vi "Turn To Angle Teleop.vi"(8 "Z Axis":dbl, 9 "PID gains":T1={"proportional gain (Kc)"=0.035, "integral time (Ti, min)"=0.0, "derivative time (Td, min)"=0.0018}, 10 "POV":i16, 11 "output range":cluster{"output high":dbl, "output low":dbl}={"output high"=1.0, "output low"=-1.0}) -> (2 "Adjustment Voltage":dbl)   [LabVIEW 2018]
uses:
  <vilib>/addons/control/pid/pid.llb/PID (DBL).vi
  <vilib>/addons/control/pid/NI_PID_pid.lvlib
panel:
  # ".0202"
  # "0"
  # ".0032150"
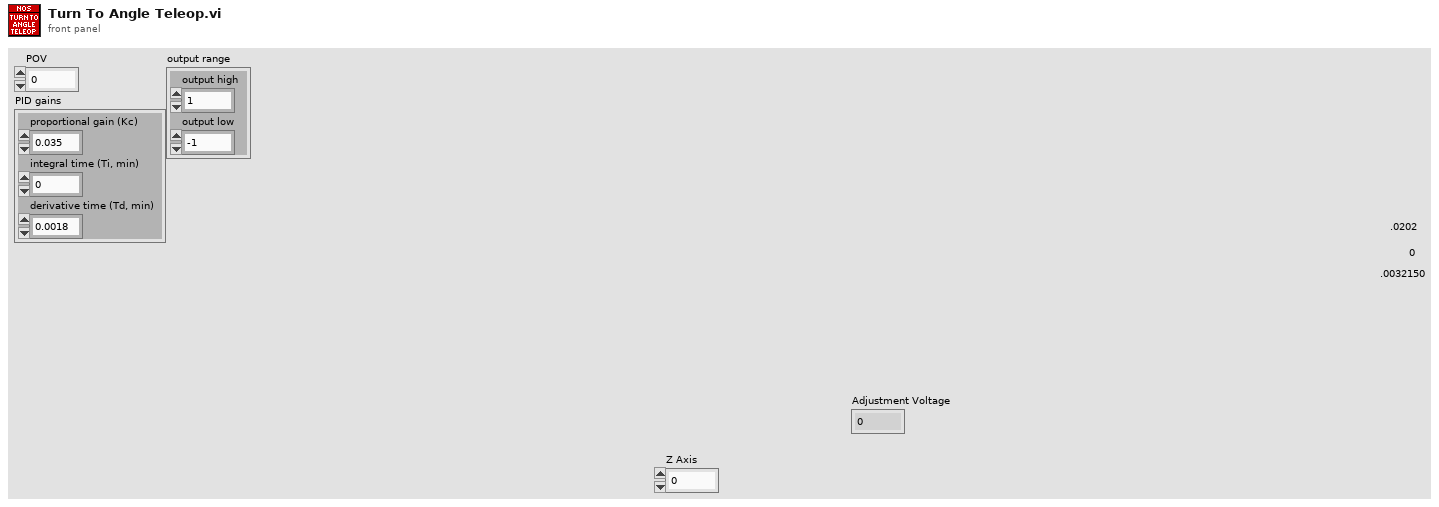
[diagram p1: front panel]
types:
  T1 = cluster{"proportional gain (Kc)":dbl, "integral time (Ti, min)":dbl, "derivative time (Td, min)":dbl}
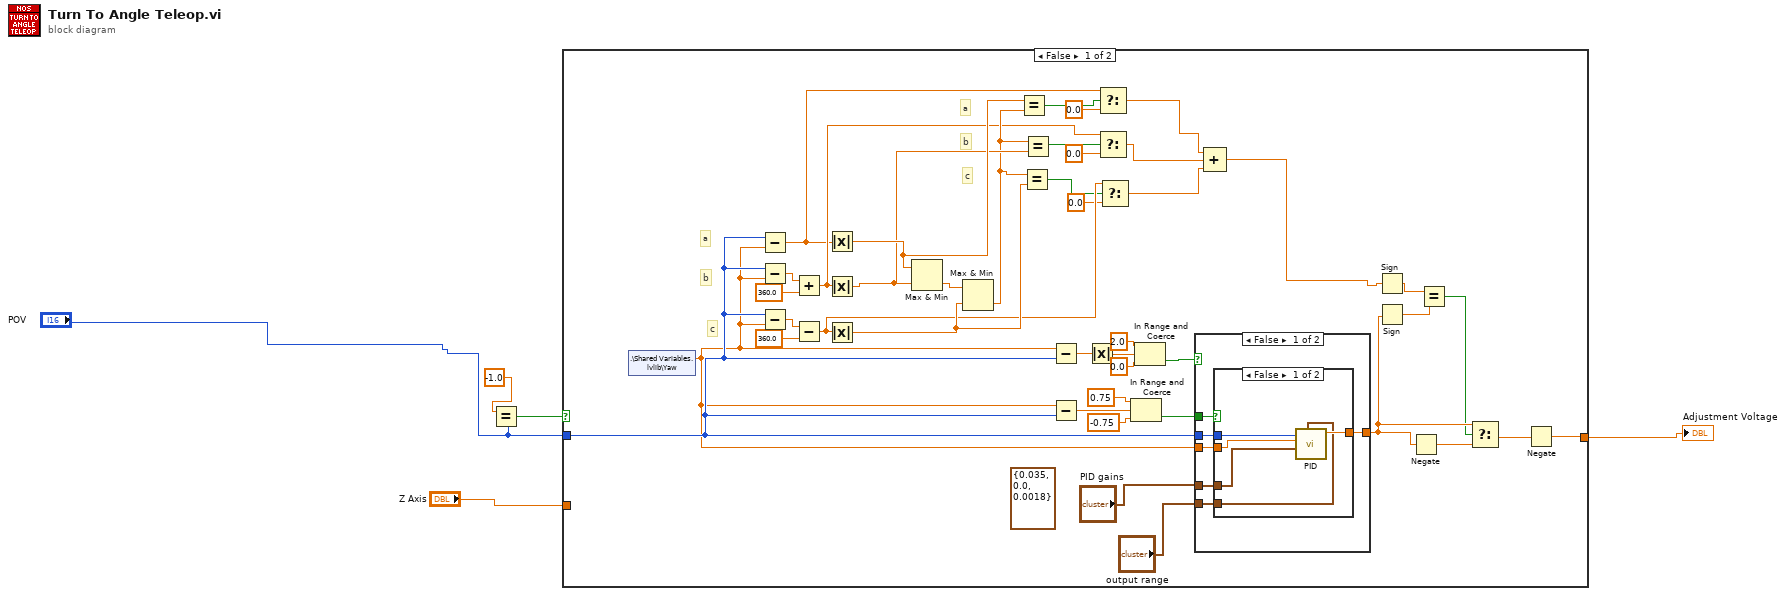
[diagram p0: block diagram]
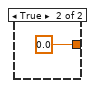
[diagram p2: hidden frame]
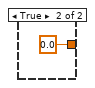
[diagram p3: hidden frame]
diagram:
  n1 = Equal?(x=-1.0, y="POV") -> (x = y?=w1:bool)
  n2 = case shown="False" w1 {
    tunnel: "POV" -> [w34 _]
    tunnel: [w8 w61] -> w4
    tunnel: "Z Axis" -> [_ w61]
    frame False {
      (unwired) T1 {"proportional gain (Kc)"=0.035, "integral time (Ti, min)"=0.0, "derivative time (Td, min)"=0.0018} ("PID gains")
      # "c"
      # "b"
      # "a"
      # "c"
      # "b"
      # "a"
      n3 = shared-variable ".\\Shared Variables.lvlib\\Yaw"() -> (w33:dbl)  [unwired: 1 in, 1 out]
      n4 = Subtract(x=w34, y=w33) -> (x-y=w25:dbl)
      n5 = Subtract(x=w34, y=w33) -> (x-y=w38:dbl)
      n6 = Subtract(x=w34, y=w33) -> (x-y=w36:dbl)
      n7 = Add(x=w38, y=360.0) -> (x+y=w26:dbl)
      n8 = Subtract(x=w36, y=360.0) -> (x-y=w24:dbl)
      n9 = Absolute Value(x=w25) -> (abs(x)=w31:dbl)
      n10 = Absolute Value(x=w26) -> (abs(x)=w30:dbl)
      n11 = Absolute Value(x=w24) -> (abs(x)=w28:dbl)
      n12 = Max & Min(x=w31, y=w30) -> (min(x,y)=w32:dbl)  [unwired: 1 out]
      n13 = Max & Min(x=w32, y=w28) -> (min(x,y)=w29:dbl)  [unwired: 1 out]
      n14 = Equal?(x=w31, y=w29) -> (x = y?=w23:bool)
      n15 = Equal?(x=w29, y=w28) -> (x = y?=w22:bool)
      n16 = Equal?(x=w29, y=w30) -> (x = y?=w27:bool)
      n17 = Subtract(x=w33, y=w34) -> (x-y=w45:dbl)
      n18 = Subtract(x=w33, y=w34) -> (x-y=w43:dbl)
      n19 = Absolute Value(x=w45) -> (abs(x)=w44:dbl)
      n20 = Select(t=w25, s=w23, f=0.0) -> (s? t:f=w18:dbl)
      n21 = Select(t=w26, s=w27, f=0.0) -> (s? t:f=w17:dbl)
      n22 = Select(t=w24, s=w22, f=0.0) -> (s? t:f=w16:dbl)
      n23 = In Range and Coerce(upper limit=0.75, x=w43, lower limit=-0.75) -> (In Range?=w40:bool)  [unwired: 1 out]
      n24 = In Range and Coerce(upper limit=2.0, x=w44, lower limit=0.0) -> (In Range?=w39:bool)  [unwired: 1 out]
      n25 = case shown="False" w39 {
        tunnel: w33 -> [w53 _]
        tunnel: w40 -> [w50 _]
        tunnel: w34 -> [w52 _]
        tunnel: [w51 0.0 ("output")] -> w13
        tunnel: "PID gains" -> [w49 _]
        tunnel: "output range" -> [w48 _]
        frame False {
          n26 = case shown="False" w50 {
            tunnel: w53 -> [w58 _]
            tunnel: w52 -> [w56 _]
            tunnel: [w57 0.0 ("output")] -> w51
            tunnel: w49 -> [w55 _]
            tunnel: w48 -> [w54 _]
            frame False {
              n27 = call-poly <vilib>:"PID.vi"("output range"=w54, "PID gains"=w55, "process variable"=w58, "setpoint"=w56) -> ("output"=w57:dbl)  [unwired: 6 in, 1 out]
            }
            frame True {
            }
          }
        }
        frame True {
        }
      }
      n28 = Compound Arithmetic op=ADD(w18, w17, w16) -> (w14:dbl)
      n29 = Sign(1:w14) -> (0:w12:dbl)
      n30 = Sign(1:w13) -> (0:w10:dbl)
      n31 = Negate(x=w13) -> (-x=w15:dbl)
      n32 = Equal?(x=w12, y=w10) -> (x = y?=w11:bool)
      n33 = Select(t=w13, s=w11, f=w15) -> (s? t:f=w9:dbl)
      n34 = Negate(x=w9) -> (-x=w8:dbl)
    }
    frame True {
    }
  }
  "Adjustment Voltage" <- w4
